vi "配置采集卡.vi"(0 "error in":errorcluster caption="错误输入", 1 "产品系列":u16(ring) items=["USB-4000", "USB-2000/1000"], 5 "SampleRate":u32=100000 caption="SampleRate (pts/s)", 7 "通道数":u32, 9 "ChanMode":u8=1, 11 "通道选择":i16, 12 "Range":sgl=10.0) -> (4 "error out":errorcluster caption="错误输出")   [LabVIEW 2016]
uses:
  PLC-Lab/lib/gusb.dll
panel:
  # "1：单端输入。\n0：差分输入。\n     选择差分输入时，只能勾选0,2,4...这样的偶数通道。"
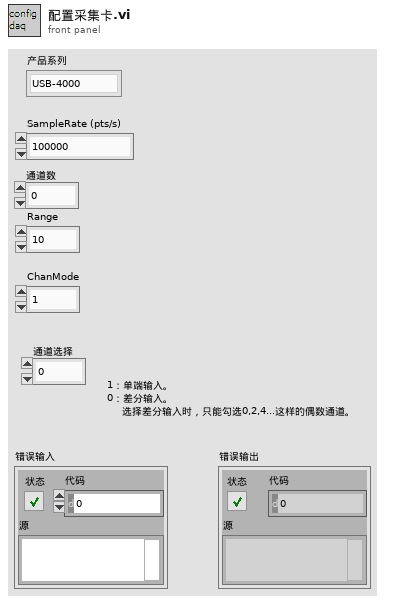
[diagram p1: front panel]
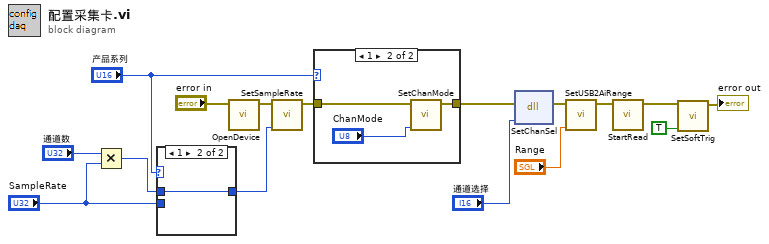
[diagram p0: block diagram]
diagram:
  n1 = Multiply(x="通道数", y="SampleRate") -> (x*y=w6:u32)
  n2 = case shown="1" "产品系列" {
    tunnel: "SampleRate" -> [w17 _]
    tunnel: [w17 w18] -> w5
    tunnel: w6 -> [_ w18]
    frame 0, Default {
    }
    frame 1 {
    }
  }
  n3 = call "OpenDevice.vi"("error in"="error in") -> ("error out"=w16:errorcluster)  [unwired: 10 in]
  n4 = call "SetSampleRate.vi"("SampleRate"=w5, "error in"=w16) -> ("error out"=w13:errorcluster)  [unwired: 9 in]
  n5 = case shown="1" "产品系列" {
    tunnel: w13 -> [w19 w22]
    tunnel: [w19 w20] -> w11
    frame 0, Default {
    }
    frame 1 {
      n6 = call "SetChanMode.vi"("ChanMode"="ChanMode", "错误输入"=w22) -> ("错误输出"=w20:errorcluster)  [unwired: 9 in]
    }
  }
  n7 = dll-call lib="E:/Camproject/2018/2018.1Labview/PLC-Lab/lib/gusb.dll" fn="SetChanSel"(error in=w11, "ChanSel"="通道选择") -> (error out=w10:errorcluster)  [unwired: 4 in, 1 out]
  n8 = call "SetUSB2AiRange.vi"("Range"="Range", "error in"=w10) -> ("error out"=w3:errorcluster)  [unwired: 9 in]
  n9 = call "StartRead.vi"("error in"=w3) -> ("error out"=w2:errorcluster)  [unwired: 10 in]
  n10 = call "SetSoftTrig.vi"("SoftTrig"=TRUE, "error in"=w2) -> ("error out"=→"error out":errorcluster)  [unwired: 9 in]
